vi "Get lasers serial nums from text file.vi"() -> (2 "Green laser serial no.":string, 3 "Blue laser serial no.":string, 4 "Error":errorcluster)   [LabVIEW 2015]
uses:
  Coherent global.vi
  <vilib>/Utility/file.llb/Read Delimited Spreadsheet (string).vi
panel:
  # "PN 04/11/2014"
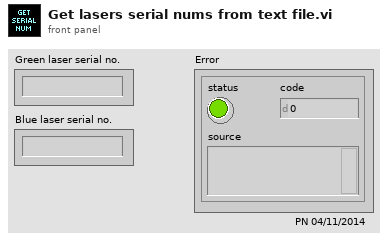
[diagram p1: front panel]
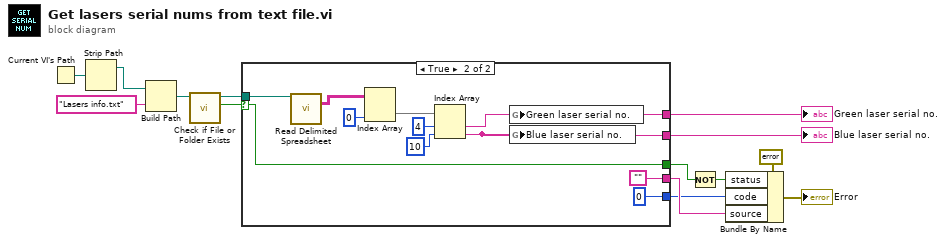
[diagram p0: block diagram]
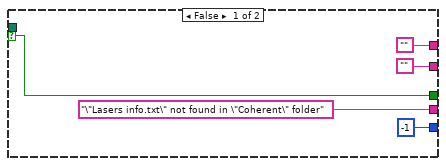
[diagram p2: hidden frame]
diagram:
  n1 = Current VI's Path() -> (path=w2:path)
  n2 = Strip Path(path=w2) -> (stripped path=w1:path)  [unwired: 1 out]
  n3 = Build Path(base path=w1, name or relative path="Lasers info.txt") -> (appended path=w3:path)
  n4 = call <vilib>:"Check if File or Folder Exists.vi"("path"=w3) -> ("file or folder exists?"=w12:bool, "dup path"=w11:path)  [unwired: 8 in, 1 out]
  n5 = case shown="True" w12 {
    selector: w12 -> [w17 w23]
    tunnel: ["" ("String") w26] -> w14
    tunnel: ["" ("String") w25] -> w13
    tunnel: w11 -> [_ w24]
    tunnel: [w17 w23] -> w9
    tunnel: ["\"Lasers info.txt\" not found in \"Coherent\" folder" ("source") "" ("source")] -> w8
    tunnel: [-1 ("code") 0 ("code")] -> w6
    frame False {
    }
    frame True {
      n6 = call-poly <vilib>:"Read Delimited Spreadsheet.vi"("file path (dialog if empty)"=w24) -> ("all rows"=w20:string[][])  [unwired: 9 in, 5 out]
      n7 = Index Array(array=w20, index (col)=0 ("disabled index (col)")) -> (element=w29:string[])  [unwired: 1 in]
      n8 = Index Array(array=w29, index #1=4 ("index"), index #2=10 ("index")) -> (element #1=w25:string, element #2=w26:string)
      n9 = global write "Coherent global.vi" "Green laser serial no."(w25) -> ()
      n10 = global write "Coherent global.vi" "Blue laser serial no."(w26) -> ()
    }
  }
  "Green laser serial no." <- w13
  "Blue laser serial no." <- w14
  n11 = Not(x=w9) -> (.not. x?=w5:bool)
  n12 = Bundle By Name(cluster=errorcluster {"status"=FALSE, "code"=0, "source"=""} ("error constant"), "status"=w5, "code"=w6, "source"=w8) -> (→"Error":errorcluster)
